vi "Read Return Message Msg.vi"(8 "error in (no error)":errorcluster, 11 "Proxy in":refnum<class "Proxy.lvclass">) -> (0 "error out":errorcluster, 2 "Proxy.lvlib:Return undeliverable Msg.lvclass":refnum<class "Return undeliverable Msg.lvclass">, 3 "Proxy out":refnum<class "Proxy.lvclass">)   [LabVIEW 2014, in "Proxy.lvlib" / "Proxy.lvclass"]
uses:
  Proxy.lvclass
  Proxy Messages/Return undeliverable Msg/Return undeliverable Msg.lvclass
  Proxy.lvclass/Proxy.ctl
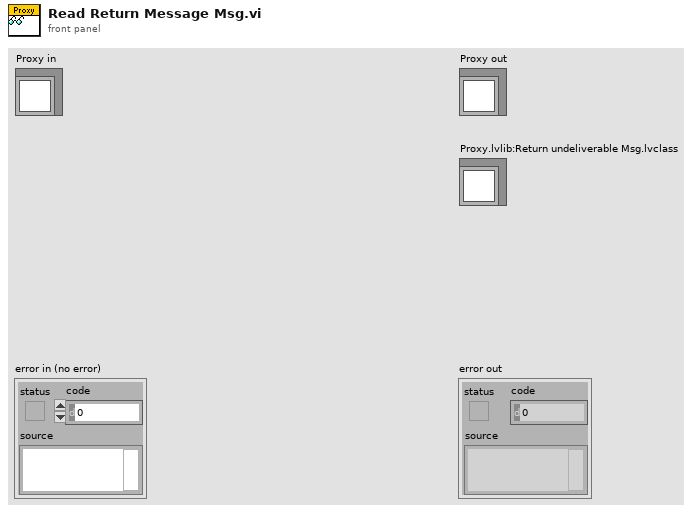
[diagram p1: front panel]
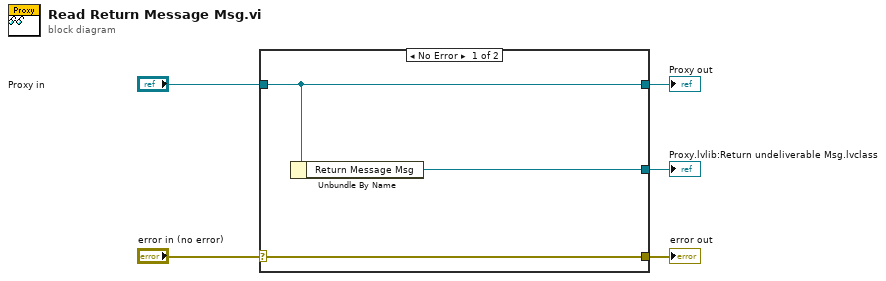
[diagram p0: block diagram]
diagram:
  n1 = case shown="No Error" "error in (no error)" {
    selector: "error in (no error)" -> [w8 w9]
    tunnel: [w8 w9] -> w4
    tunnel: [w7 w10] -> w2
    tunnel: "Proxy in" -> [w7 w10]
    tunnel: [w6 _] -> w1
    frame No Error {
      n2 = Unbundle By Name(w7) -> ("Return Message Msg"=w6:refnum<class "Return undeliverable Msg.lvclass">)
    }
    frame Error {
    }
  }
  "error out" <- w4
  "Proxy out" <- w2
  "Proxy.lvlib:Return undeliverable Msg.lvclass" <- w1
